vi "CTRE_PigeonIMU_Get6DQuaternion.vi"(8 "error in (no error)":errorcluster, 11 "PigeonIMUDevRef":T1={"DeviceStatus"={"status"=FALSE, "code"=0, "source"=""}, "Device Number"=0, "Type"=352321536, "Device ID"=0, "Handle"=0, "UsageFrame"=0, "Library Path"=path ""} {"Type" items=["CAN"=352321536, "TalonSRX"=33554432]}) -> (0 "error out":errorcluster, 2 "6D Quaternion":cluster{"W":dbl, "X":dbl, "Y":dbl, "Z":dbl}, 3 "PigeonIMUDevRef":T1={"DeviceStatus"={"status"=FALSE, "code"=0, "source"=""}, "Device Number"=0, "Type"=352321536, "Device ID"=0, "Handle"=0, "UsageFrame"=0, "Library Path"=path ""} {"Type" items=["CAN"=352321536, "TalonSRX"=33554432]})   [LabVIEW 2016]
uses:
  <vilib>/Rock Robotics/WPI/ThirdParty/Sensors/Pigeon IMU/CTRE_PigeonIMU_DeviceRef.ctl
  <vilib>/Rock Robotics/WPI/ThirdParty/Sensors/Pigeon IMU/CTRE_PigeonIMU_ConnectionType.ctl
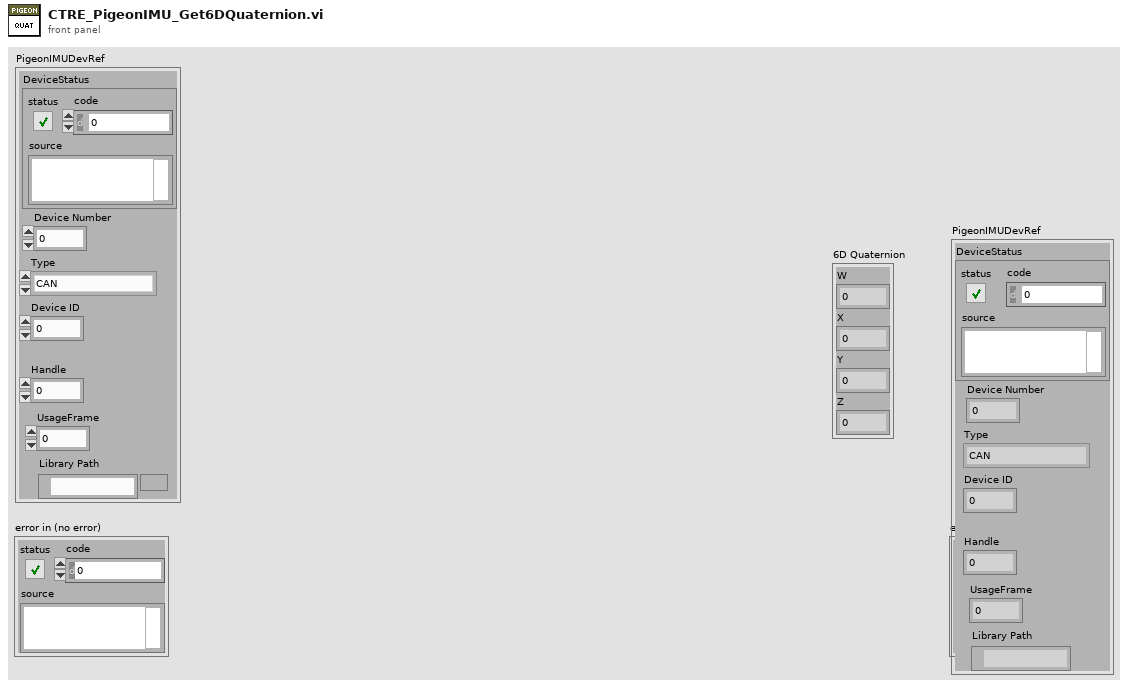
[diagram p1: front panel]
types:
  T1 = typedef "CTRE_PigeonIMU_DeviceRef.ctl" = cluster{"DeviceStatus":errorcluster, "Device Number":u8, "Type":T2, "Device ID":u32, "Handle":u64, "UsageFrame":u32, "Library Path":path}
  T2 = typedef "CTRE_PigeonIMU_ConnectionType.ctl" = u32
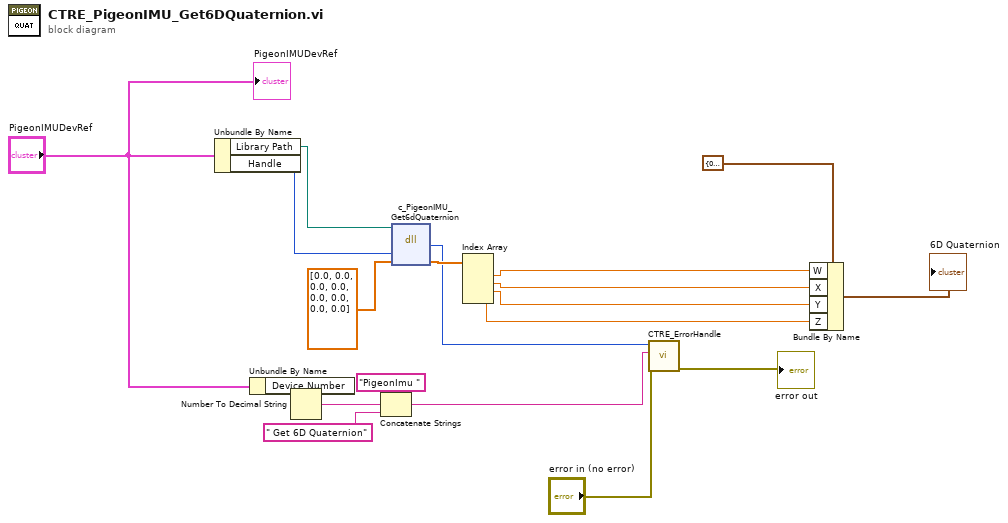
[diagram p0: block diagram]
diagram:
  n1 = Unbundle By Name("PigeonIMUDevRef") -> ("Library Path"=w10:path, "Handle"=w17:u64)
  n2 = Unbundle By Name("PigeonIMUDevRef") -> ("Device Number"=w8:u8)
  n3 = Number To Decimal String(number=w8) -> (decimal integer string=w7:string)  [unwired: 1 in]
  n4 = Concatenate Strings("PigeonImu " ("string"), w7, " Get 6D Quaternion" ("string")) -> (w4:string)
  n5 = dll-call lib="?" fn="c_PigeonIMU_Get6dQuaternion"(path in=w10, "handle"=w17, "wxyz"=dbl[] [0.0, 0.0, 0.0, 0.0, 0.0, 0.0, 0.0, 0.0]) -> ("return type"=w9:i32, "wxyz"=w16:dbl[])  [unwired: 3 in, 2 out]
  n6 = Index Array(array=w16) -> (element #1=w15:dbl, element #2=w14:dbl, element #3=w13:dbl, element #4=w12:dbl)  [unwired: 4 in]
  n7 = call <vilib>:"CTRE_ErrorHandle.vi"("error in"="error in (no error)", "origin"=w4, "code"=w9) -> ("error out"=→"error out":errorcluster)  [unwired: 8 in]
  n8 = Bundle By Name(cluster=cluster{"W":dbl, "X":dbl, "Y":dbl, "Z":dbl} {"W"=0.0, "X"=0.0, "Y"=0.0, "Z"=0.0} ("6D Quaternian"), "W"=w15, "X"=w14, "Y"=w13, "Z"=w12) -> (→"6D Quaternion":cluster{"W":dbl, "X":dbl, "Y":dbl, "Z":dbl})
  "PigeonIMUDevRef" <- "PigeonIMUDevRef"
